vi "Wago Volt Rates Parameters.vi"(8 "error in (no error)":errorcluster, 10 "Voltage Adjustment Parameters":T2, 11 "Modbus Master in":refnum<class "Modbus Master.lvclass">) -> (0 "error out":errorcluster, 3 "Modbus Master out":refnum<class "Modbus Master.lvclass">)   [LabVIEW 2016]
uses:
  <vilib>/NI/Modbus Library/API/Master/Modbus Master.lvclass
  Type Definitions/Wago Voltage Adjustment Parameters.ctl
  Type Definitions/Wago Input Commands.ctl
panel:
  in  "Ring 8":T1=263 items=["fwS1Volt1"=0, "fwS1Volt2"=1, "fwS2Volt1"=2, "fwS2Volt2"=3, "fwS3Volt1"=4, "fwS3Volt2"=5, "fwS4Volt1"=6, "fwS4Volt2"=7, "fwS5Volt1"=8, "fwS5Volt2"=9, "fwS6Volt1"=10, "fwS6Volt2 "=11, "fwS7Volt1"=12, "fwS7Volt2"=13, "fwS8Volt1"=14, "fwS8Volt2"=15, "fwRoomHum"=16, "fwRoomTemp"=17, "fwAISpare1"=18, "fwAISpare2"=19, "fwSuppTemp"=20, "fwCoolTemp"=21, "fwDehumTemp"=22, "fwUnused"=23, "Bool Inputs"=24, "gwVoltRate1"=256, "gwVoltRate2"=257, "gwVoltRate3"=258, "gwVoltRate4"=259, "gwVoltRate5"=260, "gwVoltRate6"=261, "gwVoltRate7"=262, "gwVoltRate8"=263, "gwVoltWindow5/1"=264, "gwVoltWindow6/2"=265, "gwVoltWindow7/3"=266, "gwVoltWindow8/4"=267, "fwVoltSet1"=272, "fwVoltSet2"=273, "fwVoltSet3"=274, "fwVoltSet4"=275, "fwVoltSet5"=276, "fwVoltSet6"=277, "fwVoltSet7"=278, "fwVoltSet8"=279, "fwVoltRng1"=280, "fwVoltRng2"=281, "fwVoltRng3"=282, "fwVoltRng4"=283, "fwVoltRng5"=284, "fwVoltRng6"=285, "fwVoltRng7"=286, "fwVoltRng8"=287, "fwVoltPol1"=296, "fwVoltPol2"=297, "fwVoltPol3"=298, "fwVoltPol4"=299, "fwVoltPol5"=300, "fwVoltPol6"=301, "fwVoltPol7"=302, "fwVoltPol8"=303, "Rm1St1Dr1Cmd"=304, "Rm1St2Dr1Cmd"=305, "Rm1St3Dr1Cmd"=306, "Rm1St4Dr1Cmd"=307, "Rm1St5Dr1Cmd"=308, "Rm1St6Dr1Cmd"=309, "Rm1St7Dr1Cmd"=310, "Rm1St8Dr1Cmd"=311, "Rm1St1Dr2Cmd"=312, "Rm1St2Dr2Cmd"=313, "Rm1St3Dr2Cmd"=314, "Rm1St4Dr2Cmd"=315, "Rm1St5Dr2Cmd"=316, "Rm1St6Dr2Cmd"=317, "Rm1St7Dr2Cmd"=318, "Rm1St8Dr2Cmd"=319, "Rm1St1Dr3Cmd"=320, "Rm1St2Dr3Cmd"=321, "Rm1St3Dr3Cmd"=322, "Rm1St4Dr3Cmd"=323, "Rm1St5Dr3Cmd"=324, "Rm1St6Dr3Cmd"=325, "Rm1St7Dr3Cmd"=326, "Rm1St8Dr3Cmd"=327, "fwRmTempSP"=328, "fwRmHumSP"=329, "fwCoolTempSP"=330, "fwDehumTempSP"=331, "fwRmRun"=332, "fwRmOk"=333, "fwTesting"=334, "fwRmDryP"=335, "fwRmDryI"=336, "fwRmHumP"=337, "fwRmHumI"=338, "fwRmHeatP"=339, "fwRmHeatI"=340, "fwCoolTempP"=341, "fwCoolTempI"=342, "fwDehumTempP"=343, "fwDehumTempI"=344, "fwGndLeak1"=345, "fwGndLeak2"=346, "fwGndLeak3"=347, "fwGndLeak4"=348, "fwGndLeak5"=349, "fwGndLeak6"=350, "fwGndLeak7"=351, "fwGndLeak8"=352, "Rm1OpenerCmd"=353]
  in  "Ring 7":T1=262 items=["fwS1Volt1"=0, "fwS1Volt2"=1, "fwS2Volt1"=2, "fwS2Volt2"=3, "fwS3Volt1"=4, "fwS3Volt2"=5, "fwS4Volt1"=6, "fwS4Volt2"=7, "fwS5Volt1"=8, "fwS5Volt2"=9, "fwS6Volt1"=10, "fwS6Volt2 "=11, "fwS7Volt1"=12, "fwS7Volt2"=13, "fwS8Volt1"=14, "fwS8Volt2"=15, "fwRoomHum"=16, "fwRoomTemp"=17, "fwAISpare1"=18, "fwAISpare2"=19, "fwSuppTemp"=20, "fwCoolTemp"=21, "fwDehumTemp"=22, "fwUnused"=23, "Bool Inputs"=24, "gwVoltRate1"=256, "gwVoltRate2"=257, "gwVoltRate3"=258, "gwVoltRate4"=259, "gwVoltRate5"=260, "gwVoltRate6"=261, "gwVoltRate7"=262, "gwVoltRate8"=263, "gwVoltWindow5/1"=264, "gwVoltWindow6/2"=265, "gwVoltWindow7/3"=266, "gwVoltWindow8/4"=267, "fwVoltSet1"=272, "fwVoltSet2"=273, "fwVoltSet3"=274, "fwVoltSet4"=275, "fwVoltSet5"=276, "fwVoltSet6"=277, "fwVoltSet7"=278, "fwVoltSet8"=279, "fwVoltRng1"=280, "fwVoltRng2"=281, "fwVoltRng3"=282, "fwVoltRng4"=283, "fwVoltRng5"=284, "fwVoltRng6"=285, "fwVoltRng7"=286, "fwVoltRng8"=287, "fwVoltPol1"=296, "fwVoltPol2"=297, "fwVoltPol3"=298, "fwVoltPol4"=299, "fwVoltPol5"=300, "fwVoltPol6"=301, "fwVoltPol7"=302, "fwVoltPol8"=303, "Rm1St1Dr1Cmd"=304, "Rm1St2Dr1Cmd"=305, "Rm1St3Dr1Cmd"=306, "Rm1St4Dr1Cmd"=307, "Rm1St5Dr1Cmd"=308, "Rm1St6Dr1Cmd"=309, "Rm1St7Dr1Cmd"=310, "Rm1St8Dr1Cmd"=311, "Rm1St1Dr2Cmd"=312, "Rm1St2Dr2Cmd"=313, "Rm1St3Dr2Cmd"=314, "Rm1St4Dr2Cmd"=315, "Rm1St5Dr2Cmd"=316, "Rm1St6Dr2Cmd"=317, "Rm1St7Dr2Cmd"=318, "Rm1St8Dr2Cmd"=319, "Rm1St1Dr3Cmd"=320, "Rm1St2Dr3Cmd"=321, "Rm1St3Dr3Cmd"=322, "Rm1St4Dr3Cmd"=323, "Rm1St5Dr3Cmd"=324, "Rm1St6Dr3Cmd"=325, "Rm1St7Dr3Cmd"=326, "Rm1St8Dr3Cmd"=327, "fwRmTempSP"=328, "fwRmHumSP"=329, "fwCoolTempSP"=330, "fwDehumTempSP"=331, "fwRmRun"=332, "fwRmOk"=333, "fwTesting"=334, "fwRmDryP"=335, "fwRmDryI"=336, "fwRmHumP"=337, "fwRmHumI"=338, "fwRmHeatP"=339, "fwRmHeatI"=340, "fwCoolTempP"=341, "fwCoolTempI"=342, "fwDehumTempP"=343, "fwDehumTempI"=344, "fwGndLeak1"=345, "fwGndLeak2"=346, "fwGndLeak3"=347, "fwGndLeak4"=348, "fwGndLeak5"=349, "fwGndLeak6"=350, "fwGndLeak7"=351, "fwGndLeak8"=352, "Rm1OpenerCmd"=353]
  in  "Ring 6":T1=261 items=["fwS1Volt1"=0, "fwS1Volt2"=1, "fwS2Volt1"=2, "fwS2Volt2"=3, "fwS3Volt1"=4, "fwS3Volt2"=5, "fwS4Volt1"=6, "fwS4Volt2"=7, "fwS5Volt1"=8, "fwS5Volt2"=9, "fwS6Volt1"=10, "fwS6Volt2 "=11, "fwS7Volt1"=12, "fwS7Volt2"=13, "fwS8Volt1"=14, "fwS8Volt2"=15, "fwRoomHum"=16, "fwRoomTemp"=17, "fwAISpare1"=18, "fwAISpare2"=19, "fwSuppTemp"=20, "fwCoolTemp"=21, "fwDehumTemp"=22, "fwUnused"=23, "Bool Inputs"=24, "gwVoltRate1"=256, "gwVoltRate2"=257, "gwVoltRate3"=258, "gwVoltRate4"=259, "gwVoltRate5"=260, "gwVoltRate6"=261, "gwVoltRate7"=262, "gwVoltRate8"=263, "gwVoltWindow5/1"=264, "gwVoltWindow6/2"=265, "gwVoltWindow7/3"=266, "gwVoltWindow8/4"=267, "fwVoltSet1"=272, "fwVoltSet2"=273, "fwVoltSet3"=274, "fwVoltSet4"=275, "fwVoltSet5"=276, "fwVoltSet6"=277, "fwVoltSet7"=278, "fwVoltSet8"=279, "fwVoltRng1"=280, "fwVoltRng2"=281, "fwVoltRng3"=282, "fwVoltRng4"=283, "fwVoltRng5"=284, "fwVoltRng6"=285, "fwVoltRng7"=286, "fwVoltRng8"=287, "fwVoltPol1"=296, "fwVoltPol2"=297, "fwVoltPol3"=298, "fwVoltPol4"=299, "fwVoltPol5"=300, "fwVoltPol6"=301, "fwVoltPol7"=302, "fwVoltPol8"=303, "Rm1St1Dr1Cmd"=304, "Rm1St2Dr1Cmd"=305, "Rm1St3Dr1Cmd"=306, "Rm1St4Dr1Cmd"=307, "Rm1St5Dr1Cmd"=308, "Rm1St6Dr1Cmd"=309, "Rm1St7Dr1Cmd"=310, "Rm1St8Dr1Cmd"=311, "Rm1St1Dr2Cmd"=312, "Rm1St2Dr2Cmd"=313, "Rm1St3Dr2Cmd"=314, "Rm1St4Dr2Cmd"=315, "Rm1St5Dr2Cmd"=316, "Rm1St6Dr2Cmd"=317, "Rm1St7Dr2Cmd"=318, "Rm1St8Dr2Cmd"=319, "Rm1St1Dr3Cmd"=320, "Rm1St2Dr3Cmd"=321, "Rm1St3Dr3Cmd"=322, "Rm1St4Dr3Cmd"=323, "Rm1St5Dr3Cmd"=324, "Rm1St6Dr3Cmd"=325, "Rm1St7Dr3Cmd"=326, "Rm1St8Dr3Cmd"=327, "fwRmTempSP"=328, "fwRmHumSP"=329, "fwCoolTempSP"=330, "fwDehumTempSP"=331, "fwRmRun"=332, "fwRmOk"=333, "fwTesting"=334, "fwRmDryP"=335, "fwRmDryI"=336, "fwRmHumP"=337, "fwRmHumI"=338, "fwRmHeatP"=339, "fwRmHeatI"=340, "fwCoolTempP"=341, "fwCoolTempI"=342, "fwDehumTempP"=343, "fwDehumTempI"=344, "fwGndLeak1"=345, "fwGndLeak2"=346, "fwGndLeak3"=347, "fwGndLeak4"=348, "fwGndLeak5"=349, "fwGndLeak6"=350, "fwGndLeak7"=351, "fwGndLeak8"=352, "Rm1OpenerCmd"=353]
  in  "Ring 5":T1=260 items=["fwS1Volt1"=0, "fwS1Volt2"=1, "fwS2Volt1"=2, "fwS2Volt2"=3, "fwS3Volt1"=4, "fwS3Volt2"=5, "fwS4Volt1"=6, "fwS4Volt2"=7, "fwS5Volt1"=8, "fwS5Volt2"=9, "fwS6Volt1"=10, "fwS6Volt2 "=11, "fwS7Volt1"=12, "fwS7Volt2"=13, "fwS8Volt1"=14, "fwS8Volt2"=15, "fwRoomHum"=16, "fwRoomTemp"=17, "fwAISpare1"=18, "fwAISpare2"=19, "fwSuppTemp"=20, "fwCoolTemp"=21, "fwDehumTemp"=22, "fwUnused"=23, "Bool Inputs"=24, "gwVoltRate1"=256, "gwVoltRate2"=257, "gwVoltRate3"=258, "gwVoltRate4"=259, "gwVoltRate5"=260, "gwVoltRate6"=261, "gwVoltRate7"=262, "gwVoltRate8"=263, "gwVoltWindow5/1"=264, "gwVoltWindow6/2"=265, "gwVoltWindow7/3"=266, "gwVoltWindow8/4"=267, "fwVoltSet1"=272, "fwVoltSet2"=273, "fwVoltSet3"=274, "fwVoltSet4"=275, "fwVoltSet5"=276, "fwVoltSet6"=277, "fwVoltSet7"=278, "fwVoltSet8"=279, "fwVoltRng1"=280, "fwVoltRng2"=281, "fwVoltRng3"=282, "fwVoltRng4"=283, "fwVoltRng5"=284, "fwVoltRng6"=285, "fwVoltRng7"=286, "fwVoltRng8"=287, "fwVoltPol1"=296, "fwVoltPol2"=297, "fwVoltPol3"=298, "fwVoltPol4"=299, "fwVoltPol5"=300, "fwVoltPol6"=301, "fwVoltPol7"=302, "fwVoltPol8"=303, "Rm1St1Dr1Cmd"=304, "Rm1St2Dr1Cmd"=305, "Rm1St3Dr1Cmd"=306, "Rm1St4Dr1Cmd"=307, "Rm1St5Dr1Cmd"=308, "Rm1St6Dr1Cmd"=309, "Rm1St7Dr1Cmd"=310, "Rm1St8Dr1Cmd"=311, "Rm1St1Dr2Cmd"=312, "Rm1St2Dr2Cmd"=313, "Rm1St3Dr2Cmd"=314, "Rm1St4Dr2Cmd"=315, "Rm1St5Dr2Cmd"=316, "Rm1St6Dr2Cmd"=317, "Rm1St7Dr2Cmd"=318, "Rm1St8Dr2Cmd"=319, "Rm1St1Dr3Cmd"=320, "Rm1St2Dr3Cmd"=321, "Rm1St3Dr3Cmd"=322, "Rm1St4Dr3Cmd"=323, "Rm1St5Dr3Cmd"=324, "Rm1St6Dr3Cmd"=325, "Rm1St7Dr3Cmd"=326, "Rm1St8Dr3Cmd"=327, "fwRmTempSP"=328, "fwRmHumSP"=329, "fwCoolTempSP"=330, "fwDehumTempSP"=331, "fwRmRun"=332, "fwRmOk"=333, "fwTesting"=334, "fwRmDryP"=335, "fwRmDryI"=336, "fwRmHumP"=337, "fwRmHumI"=338, "fwRmHeatP"=339, "fwRmHeatI"=340, "fwCoolTempP"=341, "fwCoolTempI"=342, "fwDehumTempP"=343, "fwDehumTempI"=344, "fwGndLeak1"=345, "fwGndLeak2"=346, "fwGndLeak3"=347, "fwGndLeak4"=348, "fwGndLeak5"=349, "fwGndLeak6"=350, "fwGndLeak7"=351, "fwGndLeak8"=352, "Rm1OpenerCmd"=353]
  in  "Ring 4":T1=259 items=["fwS1Volt1"=0, "fwS1Volt2"=1, "fwS2Volt1"=2, "fwS2Volt2"=3, "fwS3Volt1"=4, "fwS3Volt2"=5, "fwS4Volt1"=6, "fwS4Volt2"=7, "fwS5Volt1"=8, "fwS5Volt2"=9, "fwS6Volt1"=10, "fwS6Volt2 "=11, "fwS7Volt1"=12, "fwS7Volt2"=13, "fwS8Volt1"=14, "fwS8Volt2"=15, "fwRoomHum"=16, "fwRoomTemp"=17, "fwAISpare1"=18, "fwAISpare2"=19, "fwSuppTemp"=20, "fwCoolTemp"=21, "fwDehumTemp"=22, "fwUnused"=23, "Bool Inputs"=24, "gwVoltRate1"=256, "gwVoltRate2"=257, "gwVoltRate3"=258, "gwVoltRate4"=259, "gwVoltRate5"=260, "gwVoltRate6"=261, "gwVoltRate7"=262, "gwVoltRate8"=263, "gwVoltWindow5/1"=264, "gwVoltWindow6/2"=265, "gwVoltWindow7/3"=266, "gwVoltWindow8/4"=267, "fwVoltSet1"=272, "fwVoltSet2"=273, "fwVoltSet3"=274, "fwVoltSet4"=275, "fwVoltSet5"=276, "fwVoltSet6"=277, "fwVoltSet7"=278, "fwVoltSet8"=279, "fwVoltRng1"=280, "fwVoltRng2"=281, "fwVoltRng3"=282, "fwVoltRng4"=283, "fwVoltRng5"=284, "fwVoltRng6"=285, "fwVoltRng7"=286, "fwVoltRng8"=287, "fwVoltPol1"=296, "fwVoltPol2"=297, "fwVoltPol3"=298, "fwVoltPol4"=299, "fwVoltPol5"=300, "fwVoltPol6"=301, "fwVoltPol7"=302, "fwVoltPol8"=303, "Rm1St1Dr1Cmd"=304, "Rm1St2Dr1Cmd"=305, "Rm1St3Dr1Cmd"=306, "Rm1St4Dr1Cmd"=307, "Rm1St5Dr1Cmd"=308, "Rm1St6Dr1Cmd"=309, "Rm1St7Dr1Cmd"=310, "Rm1St8Dr1Cmd"=311, "Rm1St1Dr2Cmd"=312, "Rm1St2Dr2Cmd"=313, "Rm1St3Dr2Cmd"=314, "Rm1St4Dr2Cmd"=315, "Rm1St5Dr2Cmd"=316, "Rm1St6Dr2Cmd"=317, "Rm1St7Dr2Cmd"=318, "Rm1St8Dr2Cmd"=319, "Rm1St1Dr3Cmd"=320, "Rm1St2Dr3Cmd"=321, "Rm1St3Dr3Cmd"=322, "Rm1St4Dr3Cmd"=323, "Rm1St5Dr3Cmd"=324, "Rm1St6Dr3Cmd"=325, "Rm1St7Dr3Cmd"=326, "Rm1St8Dr3Cmd"=327, "fwRmTempSP"=328, "fwRmHumSP"=329, "fwCoolTempSP"=330, "fwDehumTempSP"=331, "fwRmRun"=332, "fwRmOk"=333, "fwTesting"=334, "fwRmDryP"=335, "fwRmDryI"=336, "fwRmHumP"=337, "fwRmHumI"=338, "fwRmHeatP"=339, "fwRmHeatI"=340, "fwCoolTempP"=341, "fwCoolTempI"=342, "fwDehumTempP"=343, "fwDehumTempI"=344, "fwGndLeak1"=345, "fwGndLeak2"=346, "fwGndLeak3"=347, "fwGndLeak4"=348, "fwGndLeak5"=349, "fwGndLeak6"=350, "fwGndLeak7"=351, "fwGndLeak8"=352, "Rm1OpenerCmd"=353]
  in  "Ring 3":T1=258 items=["fwS1Volt1"=0, "fwS1Volt2"=1, "fwS2Volt1"=2, "fwS2Volt2"=3, "fwS3Volt1"=4, "fwS3Volt2"=5, "fwS4Volt1"=6, "fwS4Volt2"=7, "fwS5Volt1"=8, "fwS5Volt2"=9, "fwS6Volt1"=10, "fwS6Volt2 "=11, "fwS7Volt1"=12, "fwS7Volt2"=13, "fwS8Volt1"=14, "fwS8Volt2"=15, "fwRoomHum"=16, "fwRoomTemp"=17, "fwAISpare1"=18, "fwAISpare2"=19, "fwSuppTemp"=20, "fwCoolTemp"=21, "fwDehumTemp"=22, "fwUnused"=23, "Bool Inputs"=24, "gwVoltRate1"=256, "gwVoltRate2"=257, "gwVoltRate3"=258, "gwVoltRate4"=259, "gwVoltRate5"=260, "gwVoltRate6"=261, "gwVoltRate7"=262, "gwVoltRate8"=263, "gwVoltWindow5/1"=264, "gwVoltWindow6/2"=265, "gwVoltWindow7/3"=266, "gwVoltWindow8/4"=267, "fwVoltSet1"=272, "fwVoltSet2"=273, "fwVoltSet3"=274, "fwVoltSet4"=275, "fwVoltSet5"=276, "fwVoltSet6"=277, "fwVoltSet7"=278, "fwVoltSet8"=279, "fwVoltRng1"=280, "fwVoltRng2"=281, "fwVoltRng3"=282, "fwVoltRng4"=283, "fwVoltRng5"=284, "fwVoltRng6"=285, "fwVoltRng7"=286, "fwVoltRng8"=287, "fwVoltPol1"=296, "fwVoltPol2"=297, "fwVoltPol3"=298, "fwVoltPol4"=299, "fwVoltPol5"=300, "fwVoltPol6"=301, "fwVoltPol7"=302, "fwVoltPol8"=303, "Rm1St1Dr1Cmd"=304, "Rm1St2Dr1Cmd"=305, "Rm1St3Dr1Cmd"=306, "Rm1St4Dr1Cmd"=307, "Rm1St5Dr1Cmd"=308, "Rm1St6Dr1Cmd"=309, "Rm1St7Dr1Cmd"=310, "Rm1St8Dr1Cmd"=311, "Rm1St1Dr2Cmd"=312, "Rm1St2Dr2Cmd"=313, "Rm1St3Dr2Cmd"=314, "Rm1St4Dr2Cmd"=315, "Rm1St5Dr2Cmd"=316, "Rm1St6Dr2Cmd"=317, "Rm1St7Dr2Cmd"=318, "Rm1St8Dr2Cmd"=319, "Rm1St1Dr3Cmd"=320, "Rm1St2Dr3Cmd"=321, "Rm1St3Dr3Cmd"=322, "Rm1St4Dr3Cmd"=323, "Rm1St5Dr3Cmd"=324, "Rm1St6Dr3Cmd"=325, "Rm1St7Dr3Cmd"=326, "Rm1St8Dr3Cmd"=327, "fwRmTempSP"=328, "fwRmHumSP"=329, "fwCoolTempSP"=330, "fwDehumTempSP"=331, "fwRmRun"=332, "fwRmOk"=333, "fwTesting"=334, "fwRmDryP"=335, "fwRmDryI"=336, "fwRmHumP"=337, "fwRmHumI"=338, "fwRmHeatP"=339, "fwRmHeatI"=340, "fwCoolTempP"=341, "fwCoolTempI"=342, "fwDehumTempP"=343, "fwDehumTempI"=344, "fwGndLeak1"=345, "fwGndLeak2"=346, "fwGndLeak3"=347, "fwGndLeak4"=348, "fwGndLeak5"=349, "fwGndLeak6"=350, "fwGndLeak7"=351, "fwGndLeak8"=352, "Rm1OpenerCmd"=353]
  in  "Ring 2":T1=257 items=["fwS1Volt1"=0, "fwS1Volt2"=1, "fwS2Volt1"=2, "fwS2Volt2"=3, "fwS3Volt1"=4, "fwS3Volt2"=5, "fwS4Volt1"=6, "fwS4Volt2"=7, "fwS5Volt1"=8, "fwS5Volt2"=9, "fwS6Volt1"=10, "fwS6Volt2 "=11, "fwS7Volt1"=12, "fwS7Volt2"=13, "fwS8Volt1"=14, "fwS8Volt2"=15, "fwRoomHum"=16, "fwRoomTemp"=17, "fwAISpare1"=18, "fwAISpare2"=19, "fwSuppTemp"=20, "fwCoolTemp"=21, "fwDehumTemp"=22, "fwUnused"=23, "Bool Inputs"=24, "gwVoltRate1"=256, "gwVoltRate2"=257, "gwVoltRate3"=258, "gwVoltRate4"=259, "gwVoltRate5"=260, "gwVoltRate6"=261, "gwVoltRate7"=262, "gwVoltRate8"=263, "gwVoltWindow5/1"=264, "gwVoltWindow6/2"=265, "gwVoltWindow7/3"=266, "gwVoltWindow8/4"=267, "fwVoltSet1"=272, "fwVoltSet2"=273, "fwVoltSet3"=274, "fwVoltSet4"=275, "fwVoltSet5"=276, "fwVoltSet6"=277, "fwVoltSet7"=278, "fwVoltSet8"=279, "fwVoltRng1"=280, "fwVoltRng2"=281, "fwVoltRng3"=282, "fwVoltRng4"=283, "fwVoltRng5"=284, "fwVoltRng6"=285, "fwVoltRng7"=286, "fwVoltRng8"=287, "fwVoltPol1"=296, "fwVoltPol2"=297, "fwVoltPol3"=298, "fwVoltPol4"=299, "fwVoltPol5"=300, "fwVoltPol6"=301, "fwVoltPol7"=302, "fwVoltPol8"=303, "Rm1St1Dr1Cmd"=304, "Rm1St2Dr1Cmd"=305, "Rm1St3Dr1Cmd"=306, "Rm1St4Dr1Cmd"=307, "Rm1St5Dr1Cmd"=308, "Rm1St6Dr1Cmd"=309, "Rm1St7Dr1Cmd"=310, "Rm1St8Dr1Cmd"=311, "Rm1St1Dr2Cmd"=312, "Rm1St2Dr2Cmd"=313, "Rm1St3Dr2Cmd"=314, "Rm1St4Dr2Cmd"=315, "Rm1St5Dr2Cmd"=316, "Rm1St6Dr2Cmd"=317, "Rm1St7Dr2Cmd"=318, "Rm1St8Dr2Cmd"=319, "Rm1St1Dr3Cmd"=320, "Rm1St2Dr3Cmd"=321, "Rm1St3Dr3Cmd"=322, "Rm1St4Dr3Cmd"=323, "Rm1St5Dr3Cmd"=324, "Rm1St6Dr3Cmd"=325, "Rm1St7Dr3Cmd"=326, "Rm1St8Dr3Cmd"=327, "fwRmTempSP"=328, "fwRmHumSP"=329, "fwCoolTempSP"=330, "fwDehumTempSP"=331, "fwRmRun"=332, "fwRmOk"=333, "fwTesting"=334, "fwRmDryP"=335, "fwRmDryI"=336, "fwRmHumP"=337, "fwRmHumI"=338, "fwRmHeatP"=339, "fwRmHeatI"=340, "fwCoolTempP"=341, "fwCoolTempI"=342, "fwDehumTempP"=343, "fwDehumTempI"=344, "fwGndLeak1"=345, "fwGndLeak2"=346, "fwGndLeak3"=347, "fwGndLeak4"=348, "fwGndLeak5"=349, "fwGndLeak6"=350, "fwGndLeak7"=351, "fwGndLeak8"=352, "Rm1OpenerCmd"=353]
  in  "Ring":T1=256 items=["fwS1Volt1"=0, "fwS1Volt2"=1, "fwS2Volt1"=2, "fwS2Volt2"=3, "fwS3Volt1"=4, "fwS3Volt2"=5, "fwS4Volt1"=6, "fwS4Volt2"=7, "fwS5Volt1"=8, "fwS5Volt2"=9, "fwS6Volt1"=10, "fwS6Volt2 "=11, "fwS7Volt1"=12, "fwS7Volt2"=13, "fwS8Volt1"=14, "fwS8Volt2"=15, "fwRoomHum"=16, "fwRoomTemp"=17, "fwAISpare1"=18, "fwAISpare2"=19, "fwSuppTemp"=20, "fwCoolTemp"=21, "fwDehumTemp"=22, "fwUnused"=23, "Bool Inputs"=24, "gwVoltRate1"=256, "gwVoltRate2"=257, "gwVoltRate3"=258, "gwVoltRate4"=259, "gwVoltRate5"=260, "gwVoltRate6"=261, "gwVoltRate7"=262, "gwVoltRate8"=263, "gwVoltWindow5/1"=264, "gwVoltWindow6/2"=265, "gwVoltWindow7/3"=266, "gwVoltWindow8/4"=267, "fwVoltSet1"=272, "fwVoltSet2"=273, "fwVoltSet3"=274, "fwVoltSet4"=275, "fwVoltSet5"=276, "fwVoltSet6"=277, "fwVoltSet7"=278, "fwVoltSet8"=279, "fwVoltRng1"=280, "fwVoltRng2"=281, "fwVoltRng3"=282, "fwVoltRng4"=283, "fwVoltRng5"=284, "fwVoltRng6"=285, "fwVoltRng7"=286, "fwVoltRng8"=287, "fwVoltPol1"=296, "fwVoltPol2"=297, "fwVoltPol3"=298, "fwVoltPol4"=299, "fwVoltPol5"=300, "fwVoltPol6"=301, "fwVoltPol7"=302, "fwVoltPol8"=303, "Rm1St1Dr1Cmd"=304, "Rm1St2Dr1Cmd"=305, "Rm1St3Dr1Cmd"=306, "Rm1St4Dr1Cmd"=307, "Rm1St5Dr1Cmd"=308, "Rm1St6Dr1Cmd"=309, "Rm1St7Dr1Cmd"=310, "Rm1St8Dr1Cmd"=311, "Rm1St1Dr2Cmd"=312, "Rm1St2Dr2Cmd"=313, "Rm1St3Dr2Cmd"=314, "Rm1St4Dr2Cmd"=315, "Rm1St5Dr2Cmd"=316, "Rm1St6Dr2Cmd"=317, "Rm1St7Dr2Cmd"=318, "Rm1St8Dr2Cmd"=319, "Rm1St1Dr3Cmd"=320, "Rm1St2Dr3Cmd"=321, "Rm1St3Dr3Cmd"=322, "Rm1St4Dr3Cmd"=323, "Rm1St5Dr3Cmd"=324, "Rm1St6Dr3Cmd"=325, "Rm1St7Dr3Cmd"=326, "Rm1St8Dr3Cmd"=327, "fwRmTempSP"=328, "fwRmHumSP"=329, "fwCoolTempSP"=330, "fwDehumTempSP"=331, "fwRmRun"=332, "fwRmOk"=333, "fwTesting"=334, "fwRmDryP"=335, "fwRmDryI"=336, "fwRmHumP"=337, "fwRmHumI"=338, "fwRmHeatP"=339, "fwRmHeatI"=340, "fwCoolTempP"=341, "fwCoolTempI"=342, "fwDehumTempP"=343, "fwDehumTempI"=344, "fwGndLeak1"=345, "fwGndLeak2"=346, "fwGndLeak3"=347, "fwGndLeak4"=348, "fwGndLeak5"=349, "fwGndLeak6"=350, "fwGndLeak7"=351, "fwGndLeak8"=352, "Rm1OpenerCmd"=353]
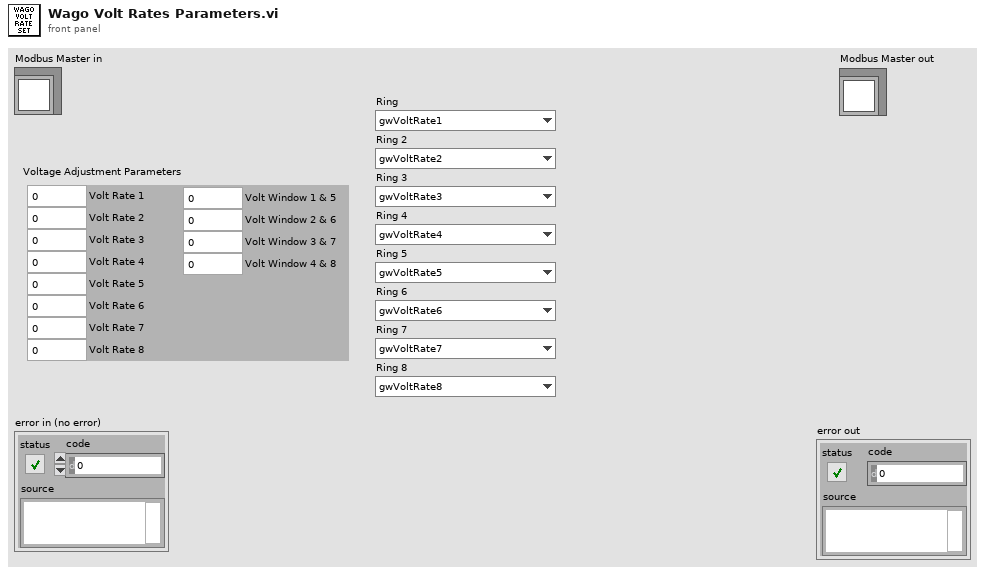
[diagram p1: front panel]
types:
  T1 = typedef "Wago Input Commands.ctl" = u16
  T2 = typedef "Wago Voltage Adjustment Parameters.ctl" = cluster{"Volt Rate 1":u16, "Volt Rate 2":u16, "Volt Rate 3":u16, "Volt Rate 4":u16, "Volt Rate 5":u16, "Volt Rate 6":u16, "Volt Rate 7":u16, "Volt Rate 8":u16, "Volt Window 1 & 5":u16, "Volt Window 2 & 6":u16, "Volt Window 3 & 7 ":u16, "Volt Window 4 & 8":u16}
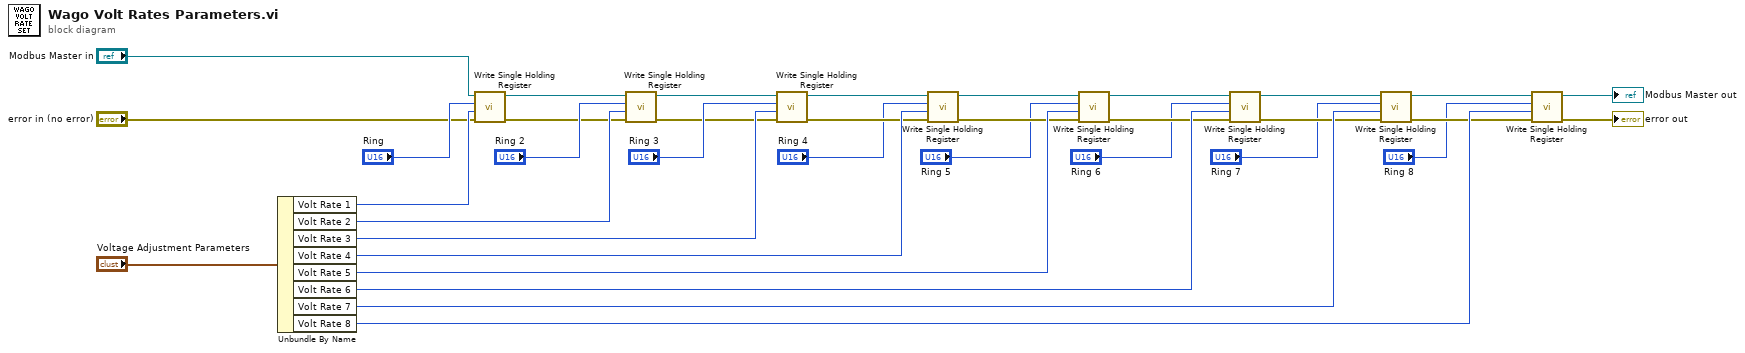
[diagram p0: block diagram]
diagram:
  n1 = Unbundle By Name("Voltage Adjustment Parameters") -> ("Volt Rate 1"=w5:u16, "Volt Rate 2"=w9:u16, "Volt Rate 3"=w28:u16, "Volt Rate 4"=w29:u16, "Volt Rate 5"=w30:u16, "Volt Rate 6"=w31:u16, "Volt Rate 7"=w32:u16, "Volt Rate 8"=w33:u16)
  n2 = call-dynamic "Write Single Holding Register.vi"("error in"="error in (no error)", "register to write"=w5, "address"="Ring", "Modbus master in"="Modbus Master in") -> ("error out"=w6:errorcluster, "Modbus master out"=w7:refnum<class "Modbus Master.lvclass">)  [unwired: 6 in]
  n3 = call-dynamic "Write Single Holding Register.vi"("error in"=w6, "register to write"=w9, "address"="Ring 2", "Modbus master in"=w7) -> ("error out"=w10:errorcluster, "Modbus master out"=w11:refnum<class "Modbus Master.lvclass">)  [unwired: 6 in]
  n4 = call-dynamic "Write Single Holding Register.vi"("error in"=w10, "register to write"=w28, "address"="Ring 3", "Modbus master in"=w11) -> ("error out"=w14:errorcluster, "Modbus master out"=w15:refnum<class "Modbus Master.lvclass">)  [unwired: 6 in]
  n5 = call-dynamic "Write Single Holding Register.vi"("error in"=w14, "register to write"=w29, "address"="Ring 4", "Modbus master in"=w15) -> ("error out"=w18:errorcluster, "Modbus master out"=w17:refnum<class "Modbus Master.lvclass">)  [unwired: 6 in]
  n6 = call-dynamic "Write Single Holding Register.vi"("error in"=w18, "register to write"=w30, "address"="Ring 5", "Modbus master in"=w17) -> ("error out"=w21:errorcluster, "Modbus master out"=w20:refnum<class "Modbus Master.lvclass">)  [unwired: 6 in]
  n7 = call-dynamic "Write Single Holding Register.vi"("error in"=w21, "register to write"=w31, "address"="Ring 6", "Modbus master in"=w20) -> ("error out"=w24:errorcluster, "Modbus master out"=w23:refnum<class "Modbus Master.lvclass">)  [unwired: 6 in]
  n8 = call-dynamic "Write Single Holding Register.vi"("error in"=w24, "register to write"=w32, "address"="Ring 7", "Modbus master in"=w23) -> ("error out"=w27:errorcluster, "Modbus master out"=w26:refnum<class "Modbus Master.lvclass">)  [unwired: 6 in]
  n9 = call-dynamic "Write Single Holding Register.vi"("error in"=w27, "register to write"=w33, "address"="Ring 8", "Modbus master in"=w26) -> ("error out"=→"error out":errorcluster, "Modbus master out"=→"Modbus Master out":refnum<class "Modbus Master.lvclass">)  [unwired: 6 in]
